vi "initLEDs.vi"() -> (0 "error out":errorcluster)   [LabVIEW 2021]
uses:
  <vilib>/rvi/eio/common/nirviEmuTemplateMethod_errors.vi
  <vilib>/eio/EIONode/EIONode.xnode
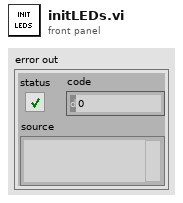
[diagram p1: front panel]
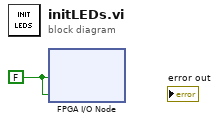
[diagram p0: block diagram]
diagram:
  w1 = FALSE ("LED0")
  n1 = xnode "FPGA I/O Node"("LED0"=w1, "LED1"=w1) -> ()  [unwired: 2 in, 2 out]
